vi "5071C.vi"(8 "error in (no error)":errorcluster caption="错误输入（无错误）", 10 "vnaPortName":refnum<visa-resource-name>, 11 "5071C输入":refnum<class "5071C.lvclass">) -> (0 "error out":errorcluster caption="错误输出", 3 "5071C输出":refnum<class "5071C.lvclass">)   [LabVIEW 2011, in "5071C.lvclass"]
uses:
  5071C.lvclass
  5071C.lvclass/5071C.ctl
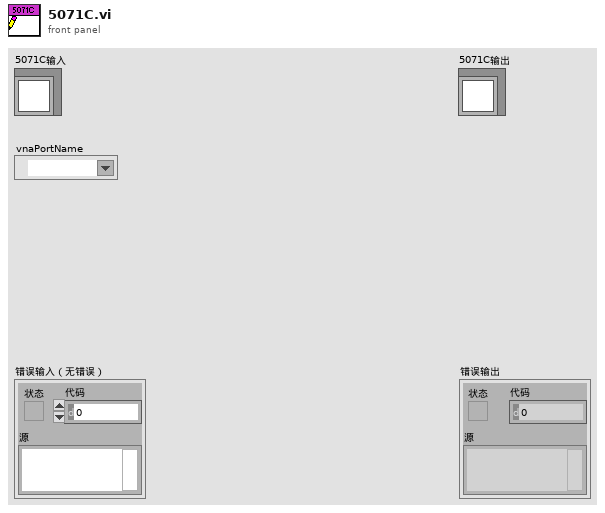
[diagram p1: front panel]
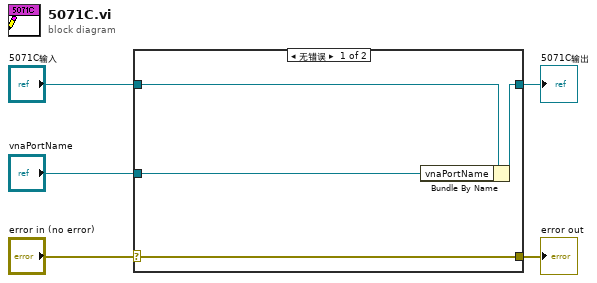
[diagram p0: block diagram]
diagram:
  n1 = case shown="无错误" "error in (no error)" {
    selector: "error in (no error)" -> [w9 w10]
    tunnel: [w9 w10] -> w4
    tunnel: [w7 w11] -> w2
    tunnel: "5071C输入" -> [w8 w11]
    tunnel: "vnaPortName" -> [w6 _]
    frame No Error {
      n2 = Bundle By Name(cluster=w8, "vnaPortName"=w6) -> (w7:refnum<class "5071C.lvclass">)
    }
    frame Error {
    }
  }
  "error out" <- w4
  "5071C输出" <- w2
